vi "FTW-CodeGen-TerminalTypeAdaption.vi"(2 "Needs Cosmetic Update on Change?":bool, 5 "FTW XNode State":T1 {"TotalCodeGens" format="CodeGens:   %04d"; "TotalAdaptToInputs" format="AdaptTerms: %04d"; "FinishedCodegen" format="%_3psec"; "ElapsedTilCodegen" format="%_3psec"; "AdaptToInputsBegin" format="%.3fmsec\n%<%D:%H:%M:%S%3u>t"}, 9 "Wired Terminals":cluster{"Type":variant, "ID":string}[](array[cluster])) -> (6 "FTW XNode State out":T1 {"TotalCodeGens" format="CodeGens:   %04d"; "TotalAdaptToInputs" format="AdaptTerms: %04d"; "FinishedCodegen" format="%_3psec"; "ElapsedTilCodegen" format="%_3psec"; "AdaptToInputsBegin" format="%.3fmsec\n%<%D:%H:%M:%S%3u>t"}, 10 "Reply":string[](array[string]))   [LabVIEW 2015]
uses:
  FTW-CodeGen-XNodeCommonState.ctl
  FTW-CodeGen-XNodeAdaptiveTerminal.ctl
  FTW-CodeGen-XNodeAdaptiveTerminal-Controller.ctl
  src/reflection/FTW-Reflection-Types.ctl
  FTW-CodeGen-XNodeAdaptiveTerminal-ControllerBehavior.ctl
  FTW-CodeGen-XNodeReplyType.ctl
  lib/FTW-KernelFilepath.vi
panel:
  # "Inputs"
  # "Outputs"
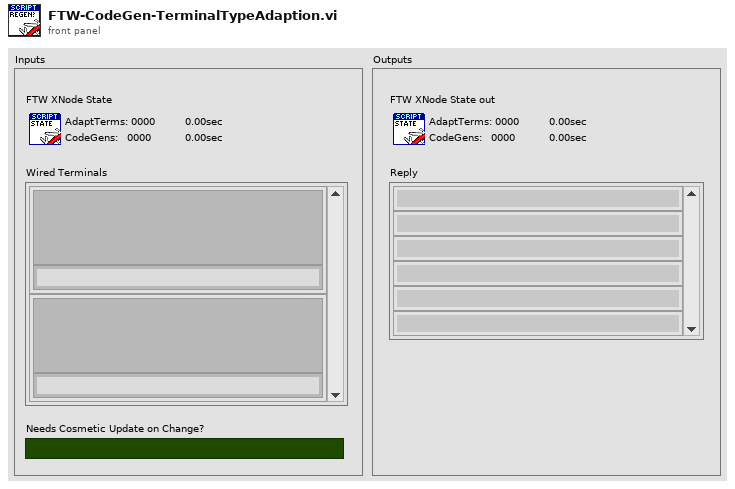
[diagram p1: front panel]
types:
  T1 = typedef "FTW-CodeGen-XNodeCommonState.ctl" = cluster{"Terms":cluster{"Name":string, "Id":string, "Type":variant, "Bounds":cluster{"Left":i32, "Top":i32, "Right":i32, "Bottom":i32}, "Input?":bool, "Required?":bool, "Recommended?":bool, "Adaptive?":bool, "Hidden?":bool, "Direction":enum32{"Auto", "Up", "Down", "Left", "Right", "Center"}, "Break Wire?":bool, "English Name":string}[], "AdaptiveTerms":T2[], "AdaptiveTerminalsOK":bool, "ForceCodeRegeneration?":bool, "LastGeneration":timestamp, "CodeGenError":errorcluster, "AdaptToInputsBegin":dbl, "ElapsedTilCodegen":dbl, "FinishedCodegen":dbl, "TotalAdaptToInputs":i32, "TotalCodeGens":i32}
  T2 = typedef "FTW-CodeGen-XNodeAdaptiveTerminal.ctl" = cluster{"Config":T3, "ID":string, "ParentIndex":i32, "Wired?":bool, "WiredTypeAllowed?":bool, "LastValidWireName":string, "LastValidWireType":T4, "Followers":i32[]}
  T3 = typedef "FTW-CodeGen-XNodeAdaptiveTerminal-Controller.ctl" = cluster{"AllowedTypes":T4[], "UnconstrainedTypeBehavior":T5, "DefaultType":variant}
  T4 = typedef "FTW-Reflection-Types.ctl" = enum16{"Unknown", "Void", "Array", "Cluster", "LVObject", "Boolean", "I8", "I16", "I32", "I64", "U8", "U16", "U32", "U64", "SGL", "DBL", "EXT", "CSG", "CDB", "CXT", "FXP", "EnumU8", "EnumU16", "EnumU32", "EnumU64", "SGLwithUnit", "DBLwithUnit", "EXTwithUnit", "CSGwithUnit", "CDBwithUnit", "CXTwithUnit", "String", "Path", "Picture", "Tag", "LVVariant", "Timestamp", "WaveformI8", "WaveformI16", "WaveformI32", "WaveformI64", "WaveformU8", "WaveformU16", "WaveformU32", "WaveformU64", "WaveformSGL", "WaveformDBL", "WaveformEXT", "WaveformCSG", "WaveformCDB", "WaveformCXT", "WaveformDigital", "WaveformUnknownType", "DigitalData", "DynamicData", "ExternalData", "FileByteStream", "TDMStream", "dotNET", "ActiveX", "VIServerReference", "VIReference", "ApplicationInstance", "Menu", "ConnectionDataSocket", "ConnectionVISA", "ConnectionBluetooth", "ConnectionIrDA", "ConnectionTCP", "ConnectionUDP", "ConnectionHTTPClient", "ConnectionFTP", "Occurrence", "Notifier", "Queue", "Rendezvous", "Semaphore", "RTFIFO", "EventPublisher", "EventRegistration", "EventCallback", "DataValueReference", "GenericClass", "GenericClassTag", "GenericClassDeepCopy", "GenericClassFlattened", "GenericClassTagFlattened", "GenericReferenceType", "WindowsRegistry", "OverloadedDatalogRef", "ReferenceUnknownType", "ByteArray", "ConPaneInterface", "FTWObject"}
  T5 = typedef "FTW-CodeGen-XNodeAdaptiveTerminal-ControllerBehavior.ctl" = enum16{"UseDefaultType", "StickyToLastValidType"}
  T6 = typedef "FTW-CodeGen-XNodeReplyType.ctl" = enum16{"NoReply", "ForceAdaptToInputs", "UpdateTerms", "GenCode", "GenCode+CosmeticUpdate"}
  T7 = cluster{"Name":string, "Id":string, "Type":variant, "Bounds":cluster{"Left":i32, "Top":i32, "Right":i32, "Bottom":i32}, "Input?":bool, "Required?":bool, "Recommended?":bool, "Adaptive?":bool, "Hidden?":bool, "Direction":enum32{"Auto", "Up", "Down", "Left", "Right", "Center"}, "Break Wire?":bool, "English Name":string}[]
  T8 = cluster{"Name":string, "Id":string, "Type":variant, "Bounds":cluster{"Left":i32, "Top":i32, "Right":i32, "Bottom":i32}, "Input?":bool, "Required?":bool, "Recommended?":bool, "Adaptive?":bool, "Hidden?":bool, "Direction":enum32{"Auto", "Up", "Down", "Left", "Right", "Center"}, "Break Wire?":bool, "English Name":string}
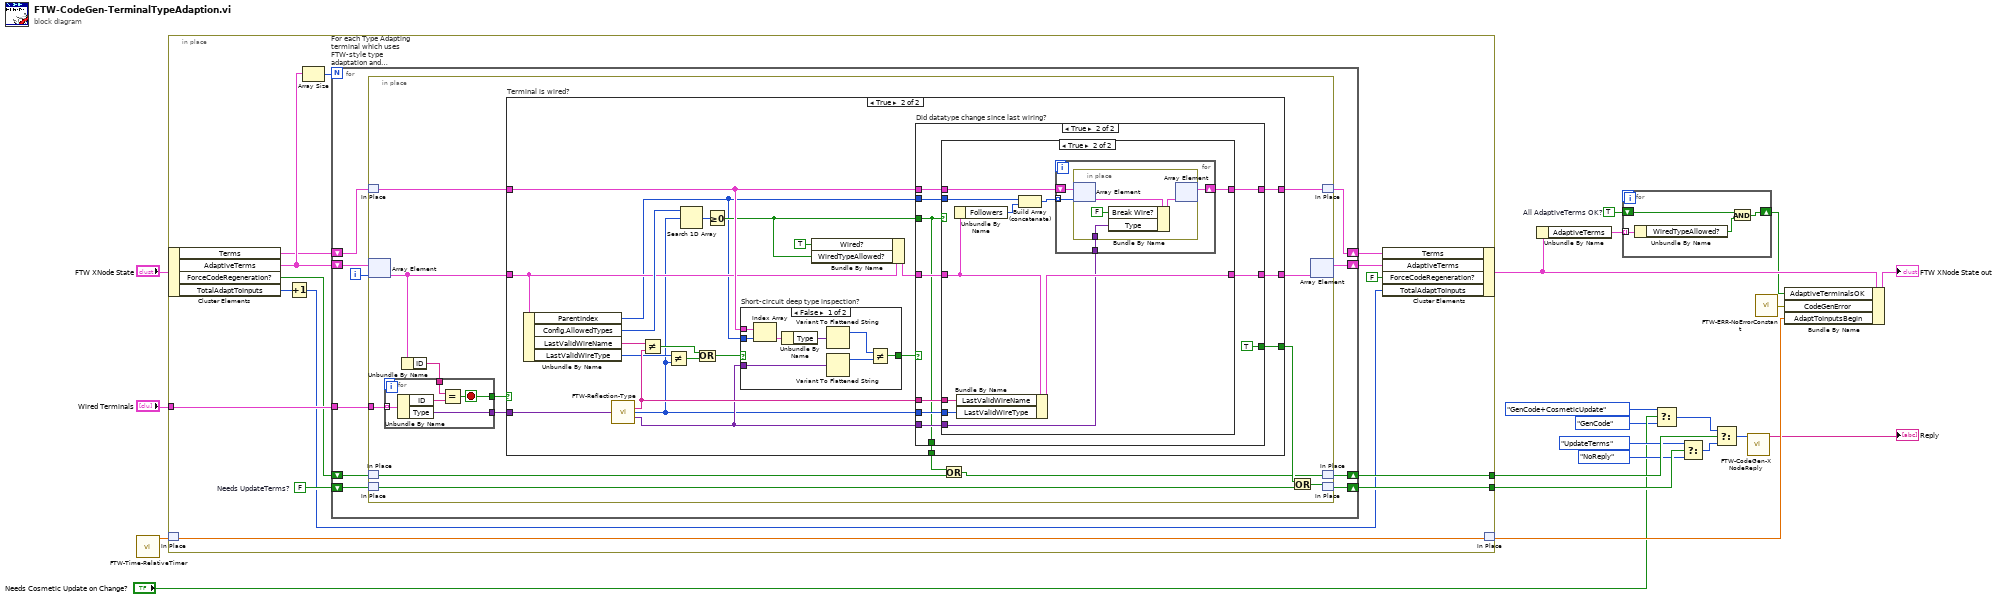
[diagram p0: block diagram]
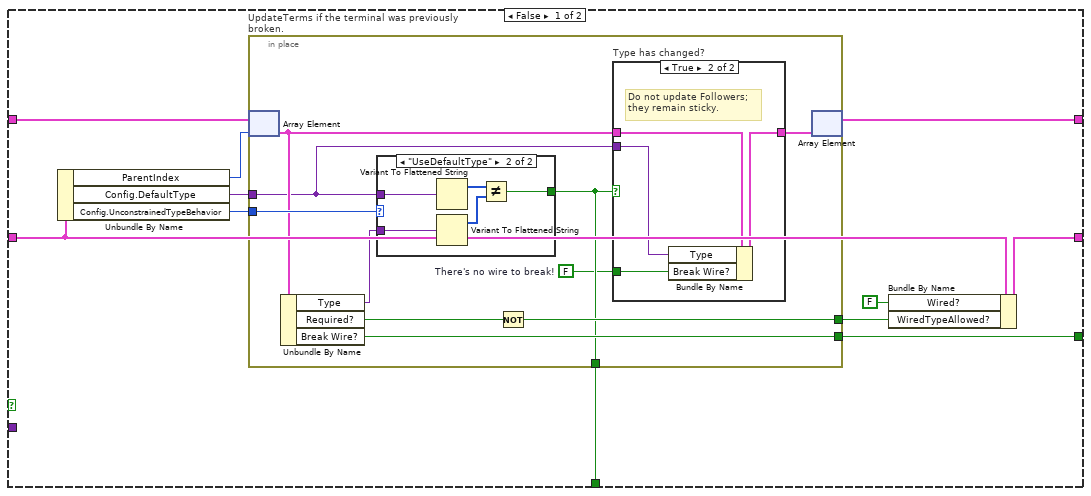
[diagram p2: hidden frame]
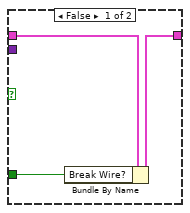
[diagram p3: hidden frame]
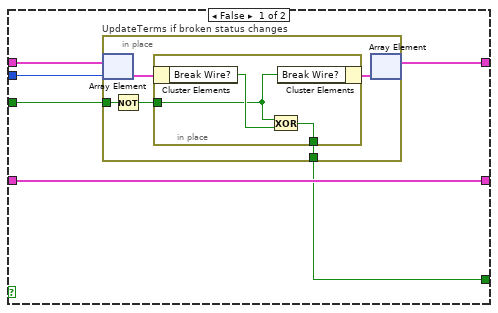
[diagram p5: hidden frame]
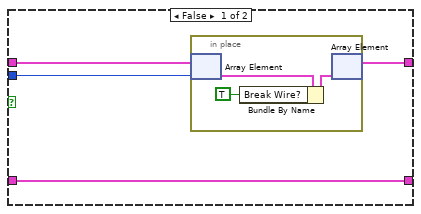
[diagram p6: hidden frame]
diagram:
  w14 = TRUE  # All AdaptiveTerms OK?
  n1 = call "FTW-Time-RelativeTimer.vi"() -> ("Current Timer Value"=w15:dbl)  [unwired: 13 in, 2 out]
  n2 = in-place {
    in-place-border: "Wired Terminals" -> [w35]
    in-place-border: [w32] -> w10
    in-place-border: [w29] -> w20
    w30 = FALSE  # Needs UpdateTerms?
    n3 = in-place-cluster #1("FTW XNode State") -> ("Terms"=w26:T7, "AdaptiveTerms"=w33:T2[], "ForceCodeRegeneration?"=w27:bool, "TotalAdaptToInputs"=w25:i32)
    n4 = in-place-match #2(w15) -> (w22:dbl)
    n5 = Increment(x=w25) -> (x+1=w24:i32)
    n6 = Array Size(array=w33) -> (size(s)=w34:i32)
    n7 = for "For each Type Adapting terminal which uses FTW-style type adaptation and propagation. The built-in type adapter and propper is simply not given enough information based on what has been (or hasn't been) wired by GenerateCode, even when the XNode\nitself knows what types should be based on a CONTROLLER-FOLLOWER relationship. Further, this enables very precise type adaptation, rather than relying on the compiler to report what could/should be bogus wiring combinations to begin with." {
      N: w34 -> [_]
      tunnel: w35 -> [w45]
      shift-right: [w42] -> w23
      shift-left: w33 -> [w44]
      shift-right: [w40] -> w28
      shift-left: w26 -> [w41]
      shift-right: [w38] -> w32
      shift-left: w27 -> [w39]
      shift-right: [w36] -> w29
      shift-left: w30 -> [w37]
      i -> [w43]
      n8 = in-place {
        in-place-border: w45 -> [w52]
        n9 = in-place-match #3(w41) -> (w56:T7)
        n10 = in-place-array #4(w44, w43) -> (w55:T2)
        n11 = in-place-match #5(w39) -> (w46:bool)
        n12 = in-place-match #6(w37) -> (w49:bool)
        n13 = Unbundle By Name(w55) -> ("ID"=w58:string)
        n14 = for {
          tunnel: [w64] -> w53
          tunnel: [w63] -> w54
          tunnel: w52 -> [w62] mode=indexing
          tunnel: w58 -> [w60]
          stop <- w63 stop-if-true
          n15 = Unbundle By Name(w62) -> ("ID"=w61:string, "Type"=w64:variant)
          n16 = Equal?(x=w60, y=w61) -> (x = y?=w63:bool)
        }
        n17 = case "Terminal is wired?" shown="True" w54 {
          tunnel: [w74 w119] -> w59
          tunnel: w55 -> [w66 w106]
          tunnel: [w68 w118] -> w57
          tunnel: w56 -> [w75 w113]
          tunnel: w53 -> [_ w112]
          tunnel: [w71 w101] -> w51
          tunnel: [w70 w98] -> w48
          frame False {
            n18 = Unbundle By Name(w66) -> ("ParentIndex"=w69:i32, "Config.DefaultType"=w73:variant, "Config.UnconstrainedTypeBehavior"=w72:T5)
            n19 = in-place "UpdateTerms if the terminal was previously broken." {
              in-place-border: w72 -> [w84]
              in-place-border: w73 -> [w76]
              in-place-border: [w83] -> w71
              in-place-border: [w81] -> w70
              in-place-border: [w82] -> w67
              w77 = FALSE  # There's no wire to break!
              n20 = in-place-array #7(w75, w69) -> (w80:T8)
              n21 = Unbundle By Name(w80) -> ("Type"=w78:variant, "Required?"=w85:bool, "Break Wire?"=w83:bool)
              n22 = case shown="\"UseDefaultType\"" w84 {
                tunnel: w76 -> [_ w95]
                tunnel: [_ w94] -> w81
                tunnel: w78 -> [_ w93]
                frame "StickyToLastValidType" {
                }
                frame "UseDefaultType" {
                  n23 = Variant To Flattened String(Variant=w95) -> (1:w96:i16[])  [unwired: 1 out]
                  n24 = Variant To Flattened String(Variant=w93) -> (1:w97:i16[])  [unwired: 1 out]
                  n25 = Not Equal?(x=w96, y=w97) -> (x != y?=w94:bool)
                }
              }
              n26 = Not(x=w85) -> (.not. x?=w82:bool)
              n27 = case "Type has changed?" shown="True" w81 {
                tunnel: w80 -> [w88 w92]
                tunnel: [w87 w91] -> w79
                tunnel: w77 -> [w86 w90]
                tunnel: w76 -> [_ w89]
                frame False {
                  n28 = Bundle By Name(cluster=w88, "Break Wire?"=w86) -> (w87:T8)
                }
                frame True {
                  # "Do not update Followers;\nthey remain sticky."
                  n29 = Bundle By Name(cluster=w92, "Type"=w89, "Break Wire?"=w90) -> (w91:T8)
                }
              }
              n30 = in-place-array #7(w79) -> (w74:T7)  [unwired: 1 out]
            }
            n31 = Bundle By Name(cluster=w66, "Wired?"=FALSE, "WiredTypeAllowed?"=w67) -> (w68:T2)
          }
          frame True {
            n32 = Unbundle By Name(w106) -> ("ParentIndex"=w99:i32, "Config.AllowedTypes"=w108:T4[], "LastValidWireName"=w114:string, "LastValidWireType"=w107:T4)
            n33 = call "FTW-Reflection-Type.vi"("Anything"=w112) -> ("Data Name"=w111:string, "LabVIEW Type"=w102:T4, "Variant Type and Value"=w110:variant)  [unwired: 12 in]
            n34 = Not Equal?(x=w114, y=w111) -> (x != y?=w116:bool)
            n35 = Not Equal?(x=w107, y=w102) -> (x != y?=w117:bool)
            n36 = Search 1D Array(1D array=w108, element=w102) -> (index of element=w109:i32)  [unwired: 1 in]
            n37 = Compound Arithmetic op=OR(w116, w117) -> (w115:bool)
            n38 = Greater Or Equal To 0?(x=w109) -> (x >= 0?=w103:bool)
            n39 = case "Short-circuit deep type inspection?" shown="False" w115 {
              selector: w115 -> [_ w177]
              tunnel: [w173 w177] -> w100
              tunnel: w110 -> [w176 _]
              tunnel: w99 -> [w171 _]
              tunnel: w113 -> [w172 _]
              frame False {
                n40 = Index Array(array=w172, index=w171) -> (element=w170:T8)
                n41 = Unbundle By Name(w170) -> ("Type"=w169:variant)
                n42 = Variant To Flattened String(Variant=w169) -> (1:w175:i16[])  [unwired: 1 out]
                n43 = Variant To Flattened String(Variant=w176) -> (1:w174:i16[])  [unwired: 1 out]
                n44 = Not Equal?(x=w175, y=w174) -> (x != y?=w173:bool)
              }
              frame True {
              }
            }
            n45 = Bundle By Name(cluster=w106, "Wired?"=TRUE, "WiredTypeAllowed?"=w103) -> (w105:T2)
            n46 = case "Did datatype change since last wiring?" shown="True" w100 {
              tunnel: w113 -> [w124 w143]
              tunnel: [w123 w142] -> w119
              tunnel: w99 -> [w120 w137]
              tunnel: w105 -> [w125 w136]
              tunnel: [w125 w141] -> w118
              tunnel: w110 -> [_ w138]
              tunnel: w102 -> [_ w140]
              tunnel: w111 -> [_ w139]
              tunnel: w103 -> [w122 w134]
              tunnel: [w121 TRUE] -> w101
              tunnel: [_ w134] -> w98
              frame False {
                n47 = in-place "UpdateTerms if broken status changes" {
                  in-place-border: w122 -> [w130]
                  in-place-border: [w126] -> w121
                  n48 = in-place-array #8(w124, w120) -> (w129:T8)
                  n49 = Not(x=w130) -> (.not. x?=w127:bool)
                  n50 = in-place {
                    in-place-border: w127 -> [w131]
                    in-place-border: [w132] -> w126
                    n51 = in-place-cluster #9(w129) -> ("Break Wire?"=w133:bool)
                    n52 = Exclusive Or(1:w133, 2:w131) -> (0:w132:bool)
                    n53 = in-place-cluster #9("Break Wire?"=w131) -> (w128:T8)
                  }
                  n54 = in-place-array #8(w128) -> (w123:T7)  [unwired: 1 out]
                }
              }
              frame True {
                n55 = case shown="True" w134 {
                  tunnel: w143 -> [w147 w160]
                  tunnel: [w145 w159] -> w142
                  tunnel: [w144 w158] -> w141
                  tunnel: w140 -> [_ w157]
                  tunnel: w139 -> [_ w156]
                  tunnel: w138 -> [_ w155]
                  tunnel: w136 -> [w144 w154]
                  tunnel: w137 -> [w146 w152]
                  frame False {
                    n56 = in-place {
                      n57 = in-place-array #10(w147, w146) -> (w150:T8)
                      n58 = Bundle By Name(cluster=w150, "Break Wire?"=TRUE) -> (w149:T8)
                      n59 = in-place-array #10(w149) -> (w145:T7)  [unwired: 1 out]
                    }
                  }
                  frame True {
                    n60 = Unbundle By Name(w154) -> ("Followers"=w153:i32[])
                    n61 = Bundle By Name(cluster=w154, "LastValidWireName"=w156, "LastValidWireType"=w157) -> (w158:T2)
                    n62 = Build Array (concatenate)(w152, w153) -> (w151:i32[])
                    n63 = for {
                      tunnel: w155 -> [w162]
                      tunnel: w151 -> [w161] mode=indexing
                      shift-right: [w163] -> w159
                      shift-left: w160 -> [w164]
                      n64 = in-place {
                        in-place-border: w162 -> [w166]
                        n65 = in-place-array #11(w164, w161) -> (w168:T8)
                        n66 = Bundle By Name(cluster=w168, "Break Wire?"=FALSE, "Type"=w166) -> (w167:T8)
                        n67 = in-place-array #11(w167) -> (w163:T7)  [unwired: 1 out]
                      }
                    }
                  }
                }
              }
            }
          }
        }
        n68 = Or(x=w48, y=w46) -> (x .or. y?=w47:bool)
        n69 = Or(x=w51, y=w49) -> (x .or. y?=w50:bool)
        n70 = in-place-array #4(w57) -> (w42:T2[])  [unwired: 1 out]
        n71 = in-place-match #3(w59) -> (w40:T7)
        n72 = in-place-match #5(w47) -> (w38:bool)
        n73 = in-place-match #6(w50) -> (w36:bool)
      }
    }
    n74 = in-place-cluster #1("Terms"=w28, "AdaptiveTerms"=w23, "ForceCodeRegeneration?"=FALSE, "TotalAdaptToInputs"=w24) -> (w18:T1)
    n75 = in-place-match #2(w22) -> (w11:dbl)
  }
  n76 = Unbundle By Name(w18) -> ("AdaptiveTerms"=w17:T2[])
  n77 = for {
    tunnel: w17 -> [w181] mode=indexing
    shift-right: [w178] -> w13
    shift-left: w14 -> [w180]
    n78 = Unbundle By Name(w181) -> ("WiredTypeAllowed?"=w179:bool)
    n79 = And(x=w180, y=w179) -> (x .and. y?=w178:bool)
  }
  n80 = Select(t=FTW-CodeGen-XNodeReplyType."GenCode+CosmeticUpdate", s="Needs Cosmetic Update on Change?", f=FTW-CodeGen-XNodeReplyType."GenCode" ("t")) -> (s? t:f=w3:T6)
  n81 = Select(t=FTW-CodeGen-XNodeReplyType."UpdateTerms" ("XNode Reply Type"), s=w20, f=FTW-CodeGen-XNodeReplyType."NoReply" ("XNode Reply Type")) -> (s? t:f=w9:T6)
  n82 = Select(t=w3, s=w10, f=w9) -> (s? t:f=w8:T6)
  n83 = call "FTW-CodeGen-XNodeReply.vi"("XNode Reply Type"=w8) -> ("Reply"=→"Reply":string[])  [unwired: 14 in]
  n84 = call "FTW-ERR-NoErrorConstant.vi"() -> ("no error"=w12:errorcluster)
  n85 = Bundle By Name(cluster=w18, "AdaptiveTerminalsOK"=w13, "CodeGenError"=w12, "AdaptToInputsBegin"=w11) -> (→"FTW XNode State out":T1)
